vi "2DpicarraywithBlank.vi"(10 "2D picture array":picture[][](array[picture])) -> (2 "2d pic array with blank":picture[][](array[picture]))   [LabVIEW 2014]
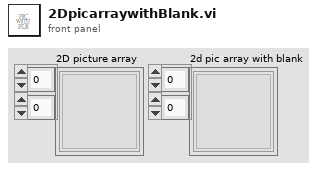
[diagram p1: front panel]
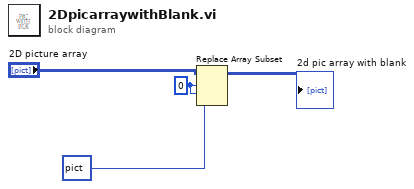
[diagram p0: block diagram]
diagram:
  w3 = 0 ("index (row)")
  n1 = Replace Array Subset(array="2D picture array", new element=picture data[5B] ("empty picture"), index (row)=w3, index (col)=w3) -> (→"2d pic array with blank":picture[][])
